vi "Linear Coefficient Calc.vi"(1 "Diameter":dbl, 2 "Power":dbl, 3 "X2":dbl, 4 "X1":dbl, 5 "T2":dbl, 6 "T1":dbl) -> (0 "K":dbl)   [LabVIEW 2017]
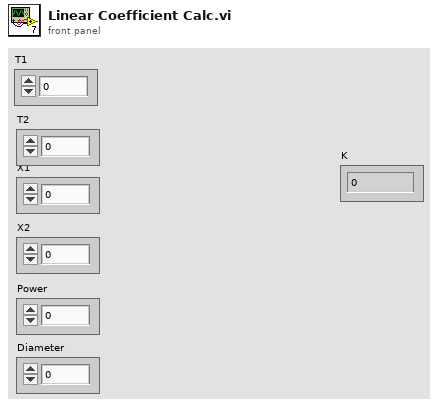
[diagram p1: front panel]
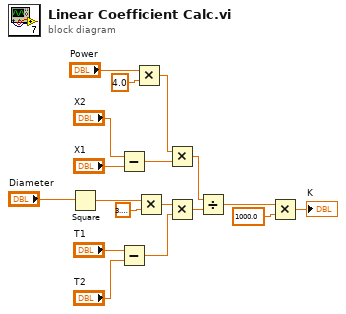
[diagram p0: block diagram]
diagram:
  n1 = Square(x="Diameter") -> (x^2=w9:dbl)
  n2 = Subtract(x="X2", y="X1") -> (x-y=w12:dbl)
  n3 = Subtract(x="T1", y="T2") -> (x-y=w4:dbl)
  n4 = Multiply(x="Power", y=4.0) -> (x*y=w13:dbl)
  n5 = Multiply(x=w9, y=3.141592653589793) -> (x*y=w5:dbl)
  n6 = Multiply(x=w13, y=w12) -> (x*y=w11:dbl)
  n7 = Multiply(x=w5, y=w4) -> (x*y=w3:dbl)
  n8 = Divide(x=w11, y=w3) -> (x/y=w2:dbl)
  n9 = Multiply(x=w2, y=1000.0) -> (x*y=→"K":dbl)
